vi "CalculateErrors.vi"   [LabVIEW 2015]
uses:
  MotorPositionGlobals.vi
  AutoVars.vi
types:
  T1 = typedef "WPI_MotorControlDeviceRef.ctl" = cluster{"DeviceStatus":errorcluster, "Type":T2, "PWM":cluster{"PWM Channel":T3, "DeadBand":T4}, "CAN":cluster{"Device Number":u8, "Control Mode":T5, "Semaphore":T6, "Max Vout":dbl, "TalonSRX Control Mode":T7}, "Invert":bool}
  T2 = typedef "WPI_MotorControlType.ctl" = enum16{"PWM", "CAN", "CANTalonSRX"}
  T3 = typedef "FPGA_DIOPWMChannel.ctl" = enum8{"PWM 0", "PWM 1", "PWM 2", "PWM 3", "PWM 4", "PWM 5", "PWM 6", "PWM 7", "PWM 8", "PWM 9", "PWM MXP 0", "PWM MXP 1", "PWM MXP 2", "PWM MXP 3", "PWM MXP 4", "PWM MXP 5", "PWM MXP 6", "PWM MXP 7", "PWM MXP 8", "PWM MXP 9", "Invalid"}
  T4 = typedef "WPI_PWMDeadband.ctl" = cluster{"Name":string, "maxPositivePwm":i32, "minPositivePwm":i32, "centerPwm":i32, "maxNegativePwm":i32, "minNegativePwm":i32, "angularRange":u16}
  T5 = typedef "WPI_CANJaguar_ControlMode.ctl" = enum8{"Percent VBus", "Current", "Speed", "Position", "Voltage"}
  T6 = typedef "Semaphore RefNum" = refnum<k1>
  T7 = typedef "WPI_CANTalonSRX_APIControlMode.ctl" = enum8{"Percent VBus", "Speed", "Position", "Slave", "Unchanged / Invalid", "Voltage Compensation", "Current", "Motion Profile"}
  T8 = typedef "WPI_CANTalonSRX_GlobalStatus.ctl" = cluster{"Applied Throttle":dbl, "Module Enabled":bool, "CAN Error":errorcluster, "Closed Loop Error":dbl, "Forward Limit Switch Closed":bool, "Reverse Limit Switch Closed":bool, "Sensor Position":dbl, "Sensor Velocity":dbl, "Current":dbl, "Sticky Fault - Over Temp":bool, "Sticky Fault - Under Voltage":bool, "Sticky Fault - Forward Limit":bool, "Sticky Fault - Reverse Limit":bool, "Sticky Fault - Forward Soft Limit":bool, "Sticky Fault - Reverse Soft Limit":bool, "Brake is Enabled":bool, "Encoder Position":dbl, "Encoder Velocity":dbl, "Encoder Index Count":dbl, "Encoder A Pin State":bool, "Encoder B Pin State":bool, "Encoder Index Pin State":bool, "Analog In":dbl, "Analog In Velocity":dbl, "Temperature (C)":dbl, "Battery Voltage":dbl, "Control 5 Is Supported":bool, "Current Profile Slot Select":dbl, "Pos Div 8":bool, "Vel Div 4":bool, "Pulse Width Position":i32, "Pulse Width Velocity":i32, "Pulse Width Rise To Rise (us)":i32, "Pulse Width Rise To Fall (us)":i32, "Mot Prof Active Is Under Run":bool, "Mot Prof Active Has Under Run":bool, "Mot Prof Active Is Last":bool, "Mot Prof Active Velocity Only":bool, "Mot Prof Active Is Valid":bool, "Mot Prof Buffer Is Full":bool, "Mot Prof Active Profile Slot Select":i32, "Mot Prof NextID":i32, "Mot Prof Count":i32, "Mot Prof Active Velocity":dbl, "Mot Prof Active Position":dbl, "Mot Prof Output Enable":i32}
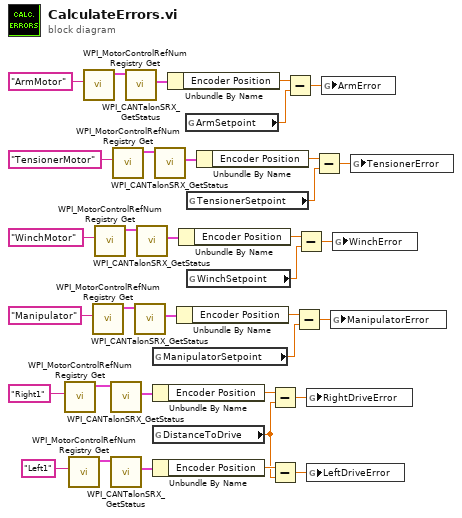
[diagram p0: block diagram]
diagram:
  n1 = call <vilib>:"WPI_MotorControlRefNum Registry Get.vi"("refnum name"="Right1") -> ("MotorControlDevRef"=w5:T1)  [unwired: 9 in, 1 out]
  n2 = call <vilib>:"WPI_MotorControlRefNum Registry Get.vi"("refnum name"="Left1") -> ("MotorControlDevRef"=w9:T1)  [unwired: 9 in, 1 out]
  n3 = call <vilib>:"WPI_MotorControlRefNum Registry Get.vi"("refnum name"="ArmMotor") -> ("MotorControlDevRef"=w33:T1)  [unwired: 9 in, 1 out]
  n4 = call <vilib>:"WPI_MotorControlRefNum Registry Get.vi"("refnum name"="Manipulator") -> ("MotorControlDevRef"=w14:T1)  [unwired: 9 in, 1 out]
  n5 = call <vilib>:"WPI_MotorControlRefNum Registry Get.vi"("refnum name"="WinchMotor") -> ("MotorControlDevRef"=w21:T1)  [unwired: 9 in, 1 out]
  n6 = call <vilib>:"WPI_CANTalonSRX_GetStatus.vi"("CAN Talon SRX Ref"=w5) -> ("Talon SRX Status"=w6:T8)  [unwired: 8 in, 2 out]
  n7 = call <vilib>:"WPI_CANTalonSRX_GetStatus.vi"("CAN Talon SRX Ref"=w9) -> ("Talon SRX Status"=w10:T8)  [unwired: 8 in, 2 out]
  n8 = call <vilib>:"WPI_MotorControlRefNum Registry Get.vi"("refnum name"="TensionerMotor") -> ("MotorControlDevRef"=w26:T1)  [unwired: 9 in, 1 out]
  n9 = call <vilib>:"WPI_CANTalonSRX_GetStatus.vi"("CAN Talon SRX Ref"=w33) -> ("Talon SRX Status"=w32:T8)  [unwired: 8 in, 2 out]
  n10 = call <vilib>:"WPI_CANTalonSRX_GetStatus.vi"("CAN Talon SRX Ref"=w14) -> ("Talon SRX Status"=w15:T8)  [unwired: 8 in, 2 out]
  n11 = call <vilib>:"WPI_CANTalonSRX_GetStatus.vi"("CAN Talon SRX Ref"=w21) -> ("Talon SRX Status"=w20:T8)  [unwired: 8 in, 2 out]
  n12 = global read "MotorPositionGlobals.vi" "ManipulatorSetpoint"() -> (w17:dbl)
  n13 = Unbundle By Name(w6) -> ("Encoder Position"=w7:dbl)
  n14 = global read "AutoVars.vi" "DistanceToDrive"() -> (w3:dbl)
  n15 = Unbundle By Name(w10) -> ("Encoder Position"=w11:dbl)
  n16 = call <vilib>:"WPI_CANTalonSRX_GetStatus.vi"("CAN Talon SRX Ref"=w26) -> ("Talon SRX Status"=w27:T8)  [unwired: 8 in, 2 out]
  n17 = Unbundle By Name(w32) -> ("Encoder Position"=w31:dbl)
  n18 = Unbundle By Name(w15) -> ("Encoder Position"=w16:dbl)
  n19 = Unbundle By Name(w20) -> ("Encoder Position"=w19:dbl)
  n20 = global read "MotorPositionGlobals.vi" "ArmSetpoint"() -> (w30:dbl)
  n21 = global read "MotorPositionGlobals.vi" "TensionerSetpoint"() -> (w29:dbl)
  n22 = global read "MotorPositionGlobals.vi" "WinchSetpoint"() -> (w18:dbl)
  n23 = Unbundle By Name(w27) -> ("Encoder Position"=w28:dbl)
  n24 = Subtract(x=w7, y=w3) -> (x-y=w1:dbl)
  n25 = Subtract(x=w11, y=w3) -> (x-y=w2:dbl)
  n26 = Subtract(x=w31, y=w30) -> (x-y=w35:dbl)
  n27 = Subtract(x=w16, y=w17) -> (x-y=w12:dbl)
  n28 = Subtract(x=w19, y=w18) -> (x-y=w23:dbl)
  n29 = global write "MotorPositionGlobals.vi" "RightDriveError"(w1) -> ()
  n30 = global write "MotorPositionGlobals.vi" "LeftDriveError"(w2) -> ()
  n31 = Subtract(x=w28, y=w29) -> (x-y=w24:dbl)
  n32 = global write "MotorPositionGlobals.vi" "ArmError"(w35) -> ()
  n33 = global write "MotorPositionGlobals.vi" "ManipulatorError"(w12) -> ()
  n34 = global write "MotorPositionGlobals.vi" "WinchError"(w23) -> ()
  n35 = global write "MotorPositionGlobals.vi" "TensionerError"(w24) -> ()
